vi "Get File Type.vi"(0 "Path":path) -> (2 "File Type":T1=enum."VIPB")   [LabVIEW 2019, in "VIPM.lvlib" / "VIPM Item.lvclass"]
uses:
  VIPM Item.lvclass
  File Type.ctl
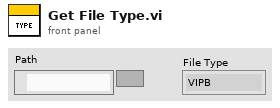
[diagram p1: front panel]
types:
  T1 = typedef "VIPM.lvlib/VIPM Item.lvclass/File Type.ctl" = enum16{"Unsupported", "VIPB", "VIPC"}
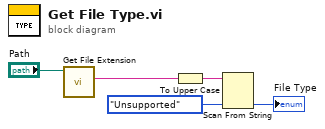
[diagram p0: block diagram]
diagram:
  n1 = call <vilib>:"Get File Extension.vi"("file"="Path") -> ("lowercase file extension"=w4:string)  [unwired: 6 in, 4 out]
  n2 = To Upper Case(1:w4) -> (0:w1:string)
  n3 = Scan From String(input string=w1, default 1=File_Type."Unsupported" ("File Type")) -> (output 1=→"File Type":T1)  [unwired: 3 in, 3 out]
